vi "Run.vi"(8 "error in":errorcluster, 11 "Client in":refnum<class "Client.lvclass">) -> (0 "error out":errorcluster, 3 "Client out":refnum<class "Client.lvclass">)   [LabVIEW 2014, in "Client.lvclass"]
uses:
  Client.lvclass
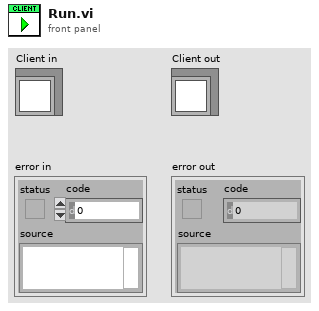
[diagram p1: front panel]
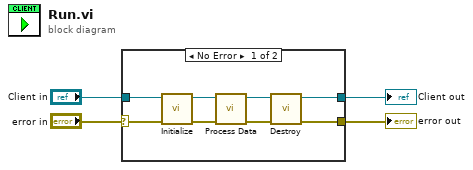
[diagram p0: block diagram]
diagram:
  n1 = case shown="No Error" "error in" {
    selector: "error in" -> [w6 w14]
    tunnel: [w5 w14] -> w3
    tunnel: [w9 w13] -> w1
    tunnel: "Client in" -> [w12 w13]
    frame No Error {
      n2 = call-dynamic "Initialize.vi"("error in"=w6, "Client in"=w12) -> ("error out"=w8:errorcluster, "Client out"=w11:refnum<class "Client.lvclass">)  [unwired: 8 in]
      n3 = call-dynamic "Process Data.vi"("error in"=w8, "Client in"=w11) -> ("error out"=w7:errorcluster, "Client out"=w10:refnum<class "Client.lvclass">)  [unwired: 8 in]
      n4 = call-dynamic "Destroy.vi"("error in"=w7, "Client in"=w10) -> ("error out"=w5:errorcluster, "Client out"=w9:refnum<class "Client.lvclass">)  [unwired: 8 in]
    }
    frame Error {
    }
  }
  "error out" <- w3
  "Client out" <- w1
